vi "CRYProbe Window Array Operation.vi"(9 "Name":string, 10 "Number":i32, 11 "sAction":string="Delete") -> ()   [LabVIEW 2013]
uses:
  Global/CRYCurve Library Global.vi
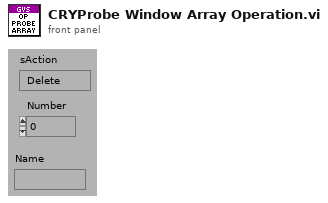
[diagram p1: front panel]
types:
  T1 = cluster{"Type Name":string, "Data Name":string, "Probe VIRef Number":i32, "Probe VIRef":refnum<vi>}[]
  T2 = cluster{"Type Name":string, "Data Name":string, "Probe VIRef Number":i32, "Probe VIRef":refnum<vi>}
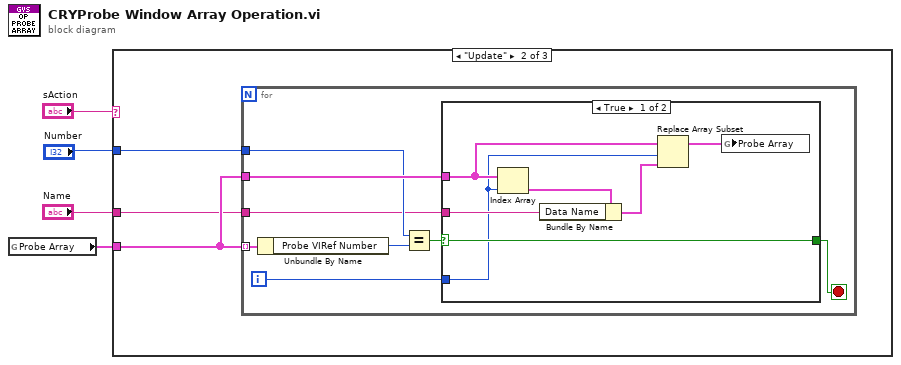
[diagram p0: block diagram]
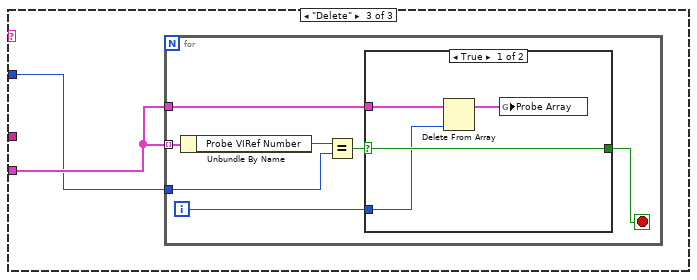
[diagram p4: hidden frame]
diagram:
  n1 = global read "CRYCurve Library Global.vi" "Probe Array"() -> (w3:T1)
  n2 = case shown="\"Update\"" "sAction" {
    tunnel: w3 -> [_ w7 w25]
    tunnel: "Name" -> [_ w6 _]
    tunnel: "Number" -> [_ w5 w24]
    frame Default {
    }
    frame "Update" {
      n3 = for {
        tunnel: w7 -> [w14] mode=indexing
        tunnel: w7 -> [w11]
        tunnel: w5 -> [w10]
        tunnel: w6 -> [w8]
        i -> [w13]
        stop <- w12 stop-if-true
        n4 = Unbundle By Name(w14) -> ("Probe VIRef Number"=w9:i32)
        n5 = Equal?(x=w10, y=w9) -> (x = y?=w15:bool)
        n6 = case shown="True" w15 {
          selector: w15 -> [w22 w23]
          tunnel: w13 -> [w16 _]
          tunnel: [w22 w23] -> w12
          tunnel: w11 -> [w19 _]
          tunnel: w8 -> [w20 _]
          frame True {
            n7 = Index Array(array=w19, index=w16) -> (element=w21:T2)
            n8 = Bundle By Name(cluster=w21, "Data Name"=w20) -> (w18:T2)
            n9 = Replace Array Subset(array=w19, new element=w18, index=w16) -> (w17:T1)
            n10 = global write "CRYCurve Library Global.vi" "Probe Array"(w17) -> ()
          }
          frame False {
          }
        }
      }
    }
    frame "Delete" {
      n11 = for {
        tunnel: w25 -> [w29] mode=indexing
        tunnel: w24 -> [w31]
        tunnel: w25 -> [w26]
        i -> [w28]
        stop <- w27 stop-if-true
        n12 = Unbundle By Name(w29) -> ("Probe VIRef Number"=w32:i32)
        n13 = Equal?(x=w32, y=w31) -> (x = y?=w30:bool)
        n14 = case shown="True" w30 {
          selector: w30 -> [w36 w37]
          tunnel: w28 -> [w33 _]
          tunnel: [w36 w37] -> w27
          tunnel: w26 -> [w34 _]
          frame True {
            n15 = Delete From Array(array=w34, index=w33) -> (array with subset deleted=w35:T1)  [unwired: 1 in, 1 out]
            n16 = global write "CRYCurve Library Global.vi" "Probe Array"(w35) -> ()
          }
          frame False {
          }
        }
      }
    }
  }
